vi "Home CYL.vi"(8 "error in":errorcluster) -> (0 "error out":errorcluster)   [LabVIEW 2021]
uses:
  Global Variables/FPGA GV.vi
  <vilib>/Utility/error.llb/Error Cluster From Error Code.vi
  <vilib>/rvi/errors/niLvFpgaAdjustHostInterfaceError.vi
  <vilib>/rvi/interface/nirviReadWriteControl/nirviReadWriteControl.xnode
  <vilib>/rvi/interface/Simulation/niFpgaSimulationCallBeginRW.vi
  NiFpgaLv.dll
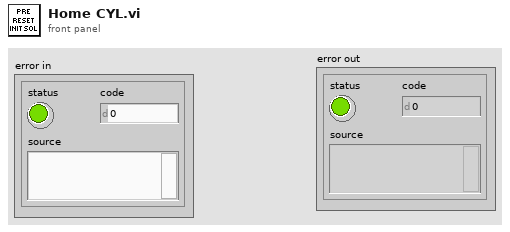
[diagram p1: front panel]
types:
  T1 = cluster{"TL_Red":bool, "TL_Orange":bool, "TL_Green":bool, "TL_Buzzer":bool, "Vaccuum ON":bool, "Vaccuum OFF":bool, "Beckhoff Data":bool, "SOL_Singling":bool, "Bowl Feeder_ ON1":bool, "Buffer 1":bool, "SOL_Pick_Place_Vertical":bool, "SOL_Tube_Feed_Agitatator":bool, "SOL_Tube_Feed_Gating_CYL":bool, "SOL_Insertion _CYL":bool, "SOL_Insertion_Clamp_CYL":bool, "SOL_Cutting_CYL":bool, "SOL_Cutting_Clamp_CYL":bool, "SOL_Insertion_Air_Nozzle":bool, "SOL_Measurement_CYL":bool, "SOL_Pick_Place_Rotary":bool, "SOL_Rejection CYL_1":bool, "SOL_Rejection CYL_2":bool, "SOL_Rejection CYL_3":bool, "SOL_Rejection CYL_4":bool, "Bowl Feeder_ON2":bool, "Linear Feeder 1":bool, "Linear Feeder 2":bool, "Buffer 2":bool, "Buffer 3":bool, "Buffer 4":bool, "Buffer 5":bool, "Buffer 6":bool}
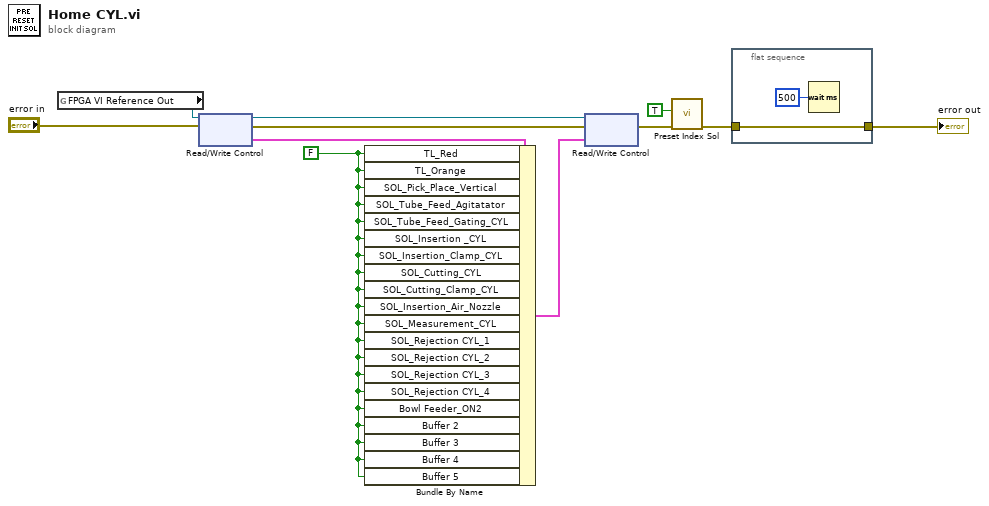
[diagram p0: block diagram]
diagram:
  w5 = FALSE ("SOL_Index_Rotary_CW")
  n1 = global read "FPGA GV.vi" "FPGA VI Reference Out"() -> (w7:refnum<k20>)
  n2 = xnode "Read/Write Control"("FPGA VI Reference In"=w7, "error in"="error in") -> ("FPGA VI Reference Out"=w11:refnum<k20>, "error out"=w10:errorcluster, "DO 1"=w9:T1)
  n3 = Bundle By Name(cluster=w9, "TL_Red"=w5, "TL_Orange"=w5, "SOL_Pick_Place_Vertical"=w5, "SOL_Tube_Feed_Agitatator"=w5, "SOL_Tube_Feed_Gating_CYL"=w5, "SOL_Insertion _CYL"=w5, "SOL_Insertion_Clamp_CYL"=w5, "SOL_Cutting_CYL"=w5, "SOL_Cutting_Clamp_CYL"=w5, "SOL_Insertion_Air_Nozzle"=w5, "SOL_Measurement_CYL"=w5, "SOL_Rejection CYL_1"=w5, "SOL_Rejection CYL_2"=w5, "SOL_Rejection CYL_3"=w5, "SOL_Rejection CYL_4"=w5, "Bowl Feeder_ON2"=w5, "Buffer 2"=w5, "Buffer 3"=w5, "Buffer 4"=w5, "Buffer 5"=w5) -> (w8:T1)
  n4 = xnode "Read/Write Control"("FPGA VI Reference In"=w11, "error in"=w10, "DO 1"=w8) -> ("error out"=w3:errorcluster)  [unwired: 1 out]
  n5 = call "Preset Index Sol.vi"("error in"=w3, "CCW?"=TRUE) -> ("error out"=w2:errorcluster)  [unwired: 9 in]
  n6 = flat-sequence {
    tunnel: w2 -> [w13]
    tunnel: [w13] -> w1
    frame #0 {
      n7 = Wait (ms)(milliseconds to wait=u32 500) -> ()  [unwired: 1 out]
    }
  }
  "error out" <- w1
